vi "Configure Message Basic.vi"() -> ()   [LabVIEW 2020, in "Yokogawa GX Series.lvlib"]
doc: "This VI sets the message writing operation."
uses:
  <instrlib>/Yokogawa GX Series/Yokogawa GX Series.lvlib
panel:
  in  "Enable Change Message (false)":bool
  in  "Enable Power-fail Message (false)":bool
  in  "Write Group (0: Common)":u16(ring) items=["Common", "Separate"]
  out "VISA resource name out":refnum<visa-resource-name>
  out "error out":errorcluster
  in  "error in (no error)":errorcluster
  in  "VISA resource name":refnum<visa-resource-name>
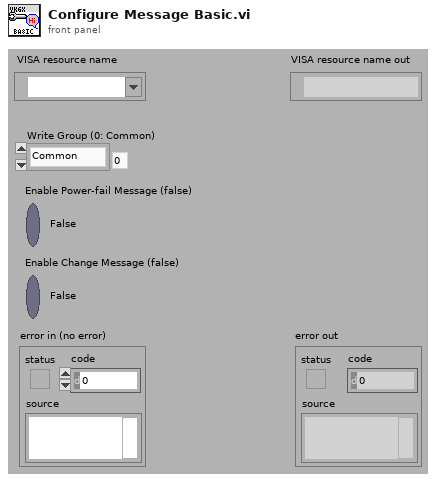
[diagram p1: front panel]
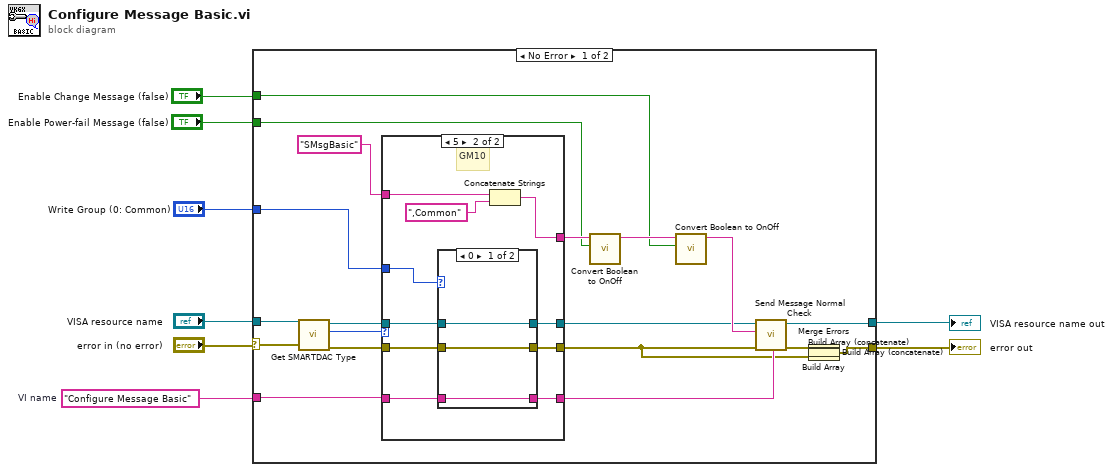
[diagram p0: block diagram]
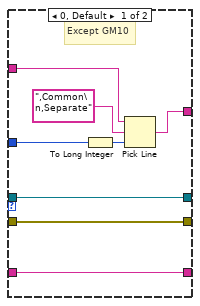
[diagram p2: hidden frame]
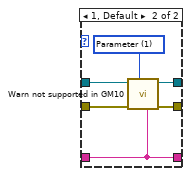
[diagram p3: hidden frame]
diagram:
  w7 = "Configure Message Basic"  # VI name
  n1 = case shown="No Error" "error in (no error)" {
    selector: "error in (no error)" -> [w18 w58]
    tunnel: "VISA resource name" -> [w28 w59]
    tunnel: w7 -> [w19 _]
    tunnel: [w20 w59] -> w6
    tunnel: [w21 w58] -> w5
    tunnel: "Write Group (0: Common)" -> [w30 _]
    tunnel: "Enable Power-fail Message (false)" -> [w24 _]
    tunnel: "Enable Change Message (false)" -> [w16 _]
    frame No Error {
      n2 = call <instrlib>:"Get SMARTDAC Type.vi"("error in (no error)"=w18, "VISA resource name"=w28) -> ("error out"=w26:errorcluster, "SMARTDAC+ Type"=w23:u16, "VISA resource name out"=w27:refnum<visa-resource-name>)  [unwired: 7 in]
      n3 = case shown="5" w23 {
        tunnel: w30 -> [w32 w40]
        tunnel: [w37 w42] -> w29
        tunnel: w27 -> [w35 w48]
        tunnel: w26 -> [w34 w47]
        tunnel: "SMsgBasic" -> [w36 w43]
        tunnel: [w35 w46] -> w14
        tunnel: [w34 w45] -> w12
        tunnel: w19 -> [w31 w41]
        tunnel: [w31 w39] -> w13
        frame 0, Default {
          # "Except GM10"
          n4 = To Long Integer(number=w32) -> (32bit integer=w33:i32)
          n5 = Pick Line(string ("")=w36, multi-line string=",Common\n,Separate", line index=w33) -> (output string=w37:string)
        }
        frame 5 {
          # "GM10"
          n6 = case shown="0" w40 {
            tunnel: w48 -> [w51 w55]
            tunnel: w47 -> [w50 w54]
            tunnel: [w51 w56] -> w46
            tunnel: [w50 w57] -> w45
            tunnel: w41 -> [w49 w52]
            tunnel: [w49 w52] -> w39
            frame 0 {
            }
            frame 1, Default {
              w53 = u16 1 items=["Command", "Parameter"] ("Kind (0: Command)")
              n7 = call <instrlib>:"Warn not supported in GM10.vi"("Source (\"\")"=w52, "Kind (0: Command)"=w53, "error in (no error)"=w54, "VISA resource name"=w55) -> ("error out"=w57:errorcluster, "VISA resource name out"=w56:refnum<visa-resource-name>)  [unwired: 6 in]
            }
          }
          n8 = Concatenate Strings(w43, ",Common") -> (w42:string)
        }
      }
      n9 = call <instrlib>:"Convert Boolean to OnOff.vi"("On/Off"=w24, "Initial String (\"\")"=w29) -> ("Resulting String"=w17:string)  [unwired: 9 in]
      n10 = call <instrlib>:"Convert Boolean to OnOff.vi"("On/Off"=w16, "Initial String (\"\")"=w17) -> ("Resulting String"=w15:string)  [unwired: 9 in]
      n11 = call <instrlib>:"Send Message Normal Check.vi"("Source (\"\")"=w13, "error in (no error)"=w12, "Send Message (\"\")"=w15, "VISA resource name"=w14) -> ("error out"=w22:errorcluster, "VISA resource name out"=w20:refnum<visa-resource-name>)  [unwired: 2 in, 4 out]
      n12 = Build Array(w22, w12) -> (w11:errorcluster[])
      n13 = Build Array (concatenate)(w11) -> (w10:errorcluster[])
      n14 = Build Array (concatenate)(w10) -> (w9:errorcluster[])
      n15 = Merge Errors(w9) -> (w21:errorcluster)
    }
    frame Error {
    }
  }
  "error out" <- w5
  "VISA resource name out" <- w6
